vi "Write line_width.vi"(8 "error in (no error)":errorcluster, 10 "line_width":i32, 11 "Field in":refnum<class "Field.lvclass">) -> (0 "error out":errorcluster, 3 "Field out":refnum<class "Field.lvclass">)   [LabVIEW 2020, in "Field.lvclass"]
uses:
  Field.lvclass
  Field.lvclass/Field.ctl
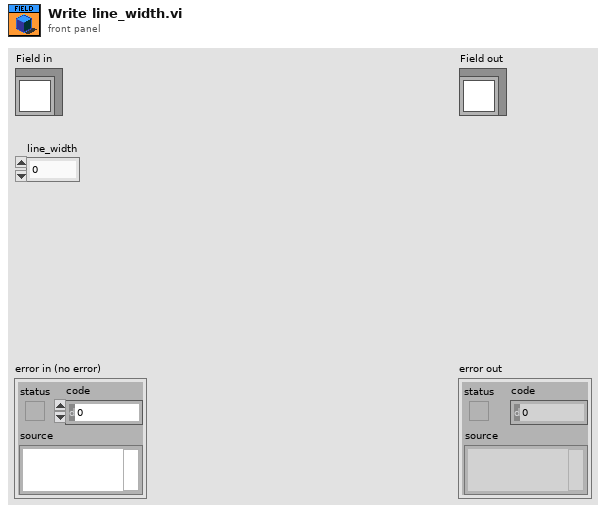
[diagram p1: front panel]
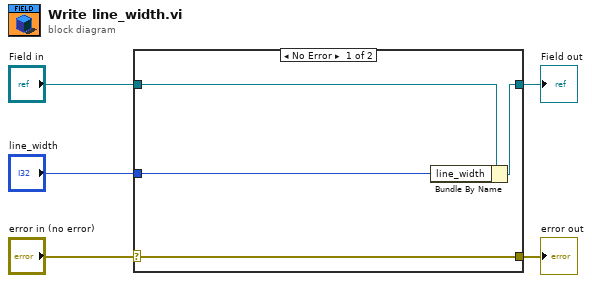
[diagram p0: block diagram]
diagram:
  n1 = case shown="No Error" "error in (no error)" {
    selector: "error in (no error)" -> [w9 w10]
    tunnel: [w9 w10] -> w4
    tunnel: [w7 w11] -> w2
    tunnel: "Field in" -> [w8 w11]
    tunnel: "line_width" -> [w6 _]
    frame No Error {
      n2 = Bundle By Name(cluster=w8, "line_width"=w6) -> (w7:refnum<class "Field.lvclass">)
    }
    frame Error {
    }
  }
  "error out" <- w4
  "Field out" <- w2
